vi "Receiver Playback from CSV.vi"() -> ()   [LabVIEW 2013]
uses:
  <vilib>/Waveform/DWDTOps.llb/DWDT Boolean Array to Digital.vi
  <vilib>/Waveform/DWDTOps.llb/DWDT Append Digital Samples.vi
  <vilib>/Waveform/DWDTOps.llb/DWDT Digital to Binary U8.vi
  <vilib>/Waveform/DWDTOps.llb/DWDT Binary U8 to Digital.vi
  <vilib>/rvi/DesktopExecutionNode/Execution/niFpgaDEN_Execute.vi
  <vilib>/rvi/DesktopExecutionNode/DesktopExecutionNode.xnode
panel:
  out "Waveform Graph":sgl[](graph)
  out "decimated array":sgl[](array[numeric])
  out "Array":sgl[](array[numeric])
  in  "file path (dialog if empty)":path=path "C:/Users/nitest/Desktop/raw_i2s.csv"
  out "sample":u32 format="%032b"
  in  "Pause":bool
  out "Digital Waveform Graph":digitalwaveform(graph)
  in  "milliseconds to wait":u32(slide)=10 scale=0.0..100.0
  in  "Graph Size":i32=100
  out "Waveform Chart":sgl(graph)
  out "Numeric":i32
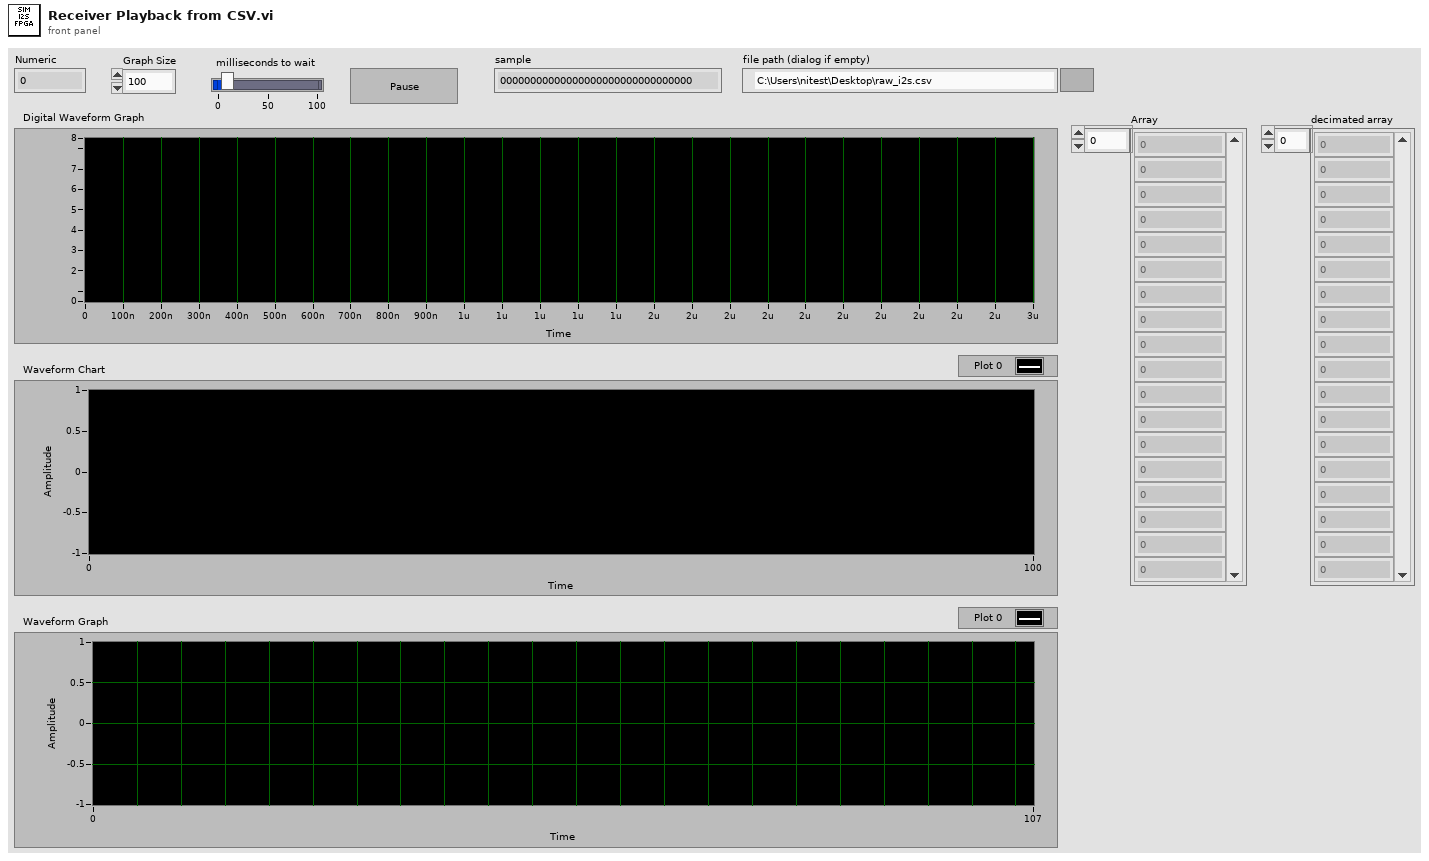
[diagram p1: front panel]
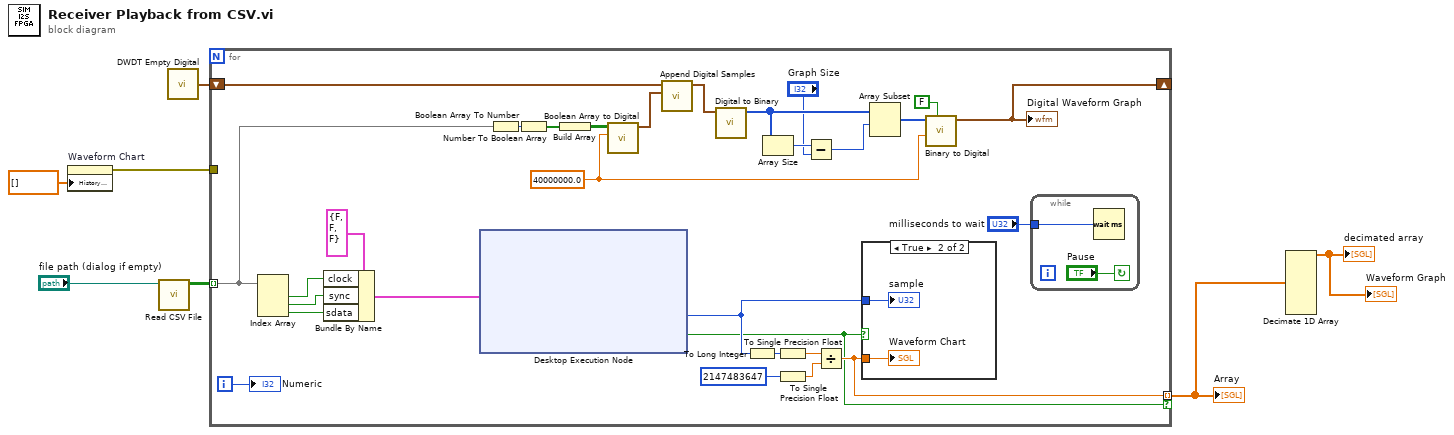
[diagram p0: block diagram]
diagram:
  n1 = property on="Waveform Chart" class="WFChart (strict)"("History Data"=sgl[] []) -> (error out=w3:errorcluster)  [unwired: 2 in, 1 out]
  n2 = call "Read CSV File.vi"("file path (dialog if empty)"="file path (dialog if empty)") -> ("signals"=w6:bool[][])  [unwired: 10 in]
  n3 = call <vilib>:"DWDT Empty Digital.vi"() -> ("digital waveform out"=w5:digitalwaveform)  [unwired: 5 in]
  n4 = for {
    tunnel: w6 -> [w14] mode=indexing
    shift-right: [w18] -> _
    shift-left: w5 -> [w27]
    tunnel: w3 -> [_]
    tunnel: [w11] -> w2 mode=indexing if=w8
    i -> [w33]
    w19 = 40000000.0 ("sample rate")
    n5 = Index Array(array=w14) -> (element #1=w28:bool, element #2=w34:bool, element #3=w35:bool)  [unwired: 3 in]
    n6 = Bundle By Name(cluster=cluster{"clock":bool, "sync":bool, "sdata":bool} {"clock"=FALSE, "sync"=FALSE, "sdata"=FALSE} ("signals in"), "clock"=w28, "sync"=w34, "sdata"=w35) -> (w10:cluster{"clock":bool, "sync":bool, "sdata":bool})
    n7 = xnode "Desktop Execution Node"("signals in"=w10) -> ("sample"=w9:u32, "output valid"=w8:bool)  [unwired: 1 in, 1 out]
    n8 = Boolean Array To Number(Boolean array=w14) -> (number=w15:u8)
    n9 = Number To Boolean Array(number=w15) -> (Boolean array=w13:bool[])
    n10 = Build Array(w13) -> (w20:bool[][])
    n11 = call-poly <vilib>:"Boolean Array to Digital.vi"("sample rate"=w19, "boolean array"=w20) -> ("digital waveform"=w17:digitalwaveform)  [unwired: 8 in, 1 out]
    n12 = call-poly <vilib>:"Append Digital Samples.vi"("digital waveform B"=w17, "digital waveform A"=w27) -> ("digital waveform out"=w16:digitalwaveform)  [unwired: 8 in, 1 out]
    n13 = call-poly <vilib>:"Digital to Binary.vi"("digital waveform"=w16) -> ("binary array"=w26:u8[])  [unwired: 9 in, 1 out]
    n14 = To Long Integer(number=w9) -> (32bit integer=w29:i32)
    n15 = Array Size(array=w26) -> (size(s)=w25:i32)
    n16 = To Single Precision Float(number=w29) -> (single precision float=w30:sgl)
    n17 = To Single Precision Float(number=2147483647) -> (single precision float=w32:sgl)
    n18 = Subtract(x=w25, y="Graph Size") -> (x-y=w24:i32)
    n19 = Divide(x=w30, y=w32) -> (x/y=w11:sgl)
    n20 = case shown="True" w8 {
      tunnel: w11 -> [_ w40]
      tunnel: w9 -> [_ w39]
      frame False {
      }
      frame True {
        "Waveform Chart" <- w40
        "sample" <- w39
      }
    }
    n21 = Array Subset(array=w26, index=w24) -> (w21:u8[])  [unwired: 1 in]
    n22 = call-poly <vilib>:"Binary to Digital.vi"("compress data (T)"=FALSE, "sample rate"=w19, "binary array"=w21) -> ("digital waveform"=w18:digitalwaveform)  [unwired: 7 in, 1 out]
    "Digital Waveform Graph" <- w18
    n23 = while {
      tunnel: "milliseconds to wait" -> [w37]
      stop <- "Pause" continue-if-true
      n24 = Wait (ms)(milliseconds to wait=w37) -> ()  [unwired: 1 out]
    }
    "Numeric" <- w33
  }
  "Array" <- w2
  n25 = Decimate 1D Array(w2) -> (→"decimated array" →"Waveform Graph":sgl[])  [unwired: 7 out]
